vi "Type Definitions.vi"() -> ()   [LabVIEW 2014]
uses:
  Labview Work/Strict Type Def Numeric.ctl
  Labview Work/Type Def Numeric.ctl
panel:
  in  "Type Def Numeric 2":dbl
  in  "Type Def Numeric":T1
  in  "Strict Type Def Numeric":T2
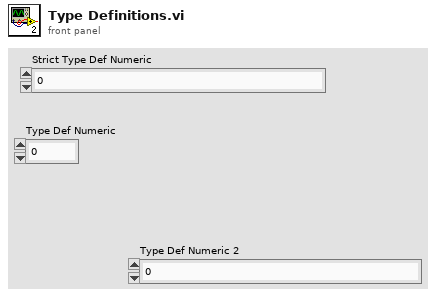
[diagram p1: front panel]
types:
  T1 = typedef "Type Def Numeric.ctl" = dbl
  T2 = typedef "Strict Type Def Numeric.ctl" = dbl
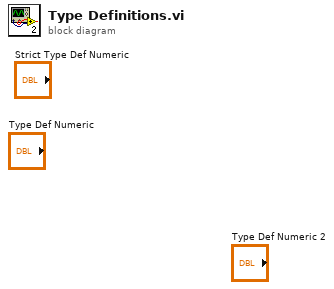
[diagram p0: block diagram]
diagram:
